vi "Current_and_Spectrum_View_new.vi"() -> ()   [LabVIEW 2009]
doc: "I. Description:\nThis example demonstrates how to perform an analog software triggered acquisition. The example allows the user to specify the triggering condition and the number of pre-trigger samples to acquire.\n \nII. Instructions for Running:\n1. Select the physical channel to correspond to where your signal is input on the DAQ device.\n2. Enter the minimum and maximum voltage ranges.\nNote: For better accuracy try to match the Input Ranges to the expected voltage level of the measured signal.\n3. Specify the rate of the sample clock. \n4. Specify the number of samples to read per iteration of the continuous input operation. These samples will then be monitored for the trigger condition. The trigger condition is determined by the parameters explained below.\n5. Specify the index of the channel that will be monitored for the requested condition. The first channel in the scan list will have an index equals to 0. It's possible to verify the name of the selected channel once the VI is run, after setting the Channel Index value.\n6. Set the triggering condition to be applied to the channel specified by the Channel Index value. The conditions created for this example are:\n\n- Rising Edge: The trigger condition is met as soon as the monitored signal falls below the Hysteresis window and then crosses past the specified Level.\n- Falling Edge: The trigger condition is met as soon as the monitored signal rises above the Hysteresis window and then crosses past the specified Level.\n- Above Level: The trigger condition is met as soon as the monitored signal is above the specified Level. \n- Below Level: The trigger condition is met as soon as the monitored signal is below the specified Level.\n- When Inside Window: The trigger condition is met as soon as the monitored signal is within the specified window.\n- When Outside Window: The trigger condition is met as soon as the monitored signal is not within the specified window.\n\n7. Set the Level value to be used by the selected condition.\n8. Set the Window Amplitude/ Hysteresis to be used by the Window/Edge conditions\n\n- The upper limit of the conditional window is calculated by adding the Window Amplitude to the condition Level.\n- The lower limit of the conditional window is calculated by subtracting the Window Amplitude from the condition Level.\n- The Hysteresis window for the Rising Edge condition is defined as Level minus the Hysteresis value. \n- The Hysteresis window for the Falling Edge condition is defined as Level plus the Hysteresis value.\n\n8. Set the number of pre-trigger samples if desired.\n\nIII. Block Diagram Steps:\n1. Create an analog input voltage channel.\n2. Find out how many channels are being used in this operation.\n3. Define the Sample Clock Rate. Additionally, define the sample mode to be continuous.\n4. Show the Channel Name of the Condition Channel.\n5. Initialize the data arrays to be used for holding successive iterations of data. This pre-allocation of memory improves the performance of the application. Refer to the VI documentation for more information.\n\nNOTE: The number of samples that meet the triggering condition is not fixed; it depends on the value of the monitored signal. This means that the number of samples to be returned by Analog Trigger Through Software (Scaled).VI may vary from one iteration to the next. In order to avoid dynamically allocating memory while filtering the data (a process that creates), this example pre-allocates arrays for the data before the acquisition starts. The arrays are initialized to the maximum number of elements expected per iteration.\n\n6. Call the Start VI to start the acquisition.\n7. Read the scaled analog input data.\nNote: The Shift Registers attached to the While Loop are used to keep track of triggering status and previous data samples (needed for pre-triggered acquisitions). \n8. Use the Analog Trigger Through Software (Scaled).VI specifically created for this example to detect the requested trigger condition through software.\n9. Show the acquired data if the trigger condition is met.\n10. Stop the loop if the trigger condition is met, an error occurs or the Stop button is pressed. \n11. Call the Clear Task VI to clear the Task.\n12. Use the popup dialog box to display an error or warning if any.\n\nIV. I/O Connections Overview:\nMake sure your signal input terminal matches the Physical Channel I/O control. For further connection information, refer to your hardware reference manual."
uses:
  <vilib>/Utility/error.llb/DialogType.ctl
  <vilib>/DAQmx/configure/timing.llb/DAQmx Timing (Sample Clock).vi
  <vilib>/DAQmx/create/channels.llb/DAQmx Create Channel (AI-Voltage-Basic).vi
  <vilib>/DAQmx/read.llb/DAQmx Read (Analog 2D DBL NChan NSamp).vi
  <vilib>/express/express analysis/Spectral/XNode/ExpressSpectralMeasurementsBlockNode.xnode
  <vilib>/express/express analysis/Spectral/Block/exnSpectralBlock spectral measurements peak poly.vi
  <vilib>/express/express analysis/Spectral/Block/exnSpectralBlock spectral measurements peak DDT.vi
  <vilib>/Utility/file.llb/Write To Spreadsheet File (DBL).vi
panel:
  in  "Save?":bool
  in  "Path":path
  in  "SAVED FILES":i32
  in  "Filename":string
  out "x/y":dbl[](array[numeric])
  out "Waveform Graph 2":dynamicdata(graph)
  out "# Pretrigger Samples\nAcquired":i32
  out "Waveform Graph":dbl[][](graph)
  out "Pre-Trigger Error Indicator":bool caption="Error Indicator\n(Indicates if trigger occurs before\npre-trigger samples were acquired)"
  in  "Pretrigger Samples":i32
  in  "Window Amplitude":dbl=0.5 caption="Window Amplitude\n/Hysteresis" step=0.10000000149011612 format="%.2p"
  out "Channel Name":string
  in  "Condition":T1(ring)=enum."Above Level"
  in  "Channel Index":i32
  in  "Level":dbl=-11.0 step=0.10000000149011612 format="%.2p"
  in  "Samples to Read":i32=40000 caption="Samples to Read per Iteration"
  in  "Maximum Value":dbl=10.0 format="%.2p"
  in  "Minimum Value":dbl=-10.0 format="%.2p"
  in  "Physical Channel":tag="Dev1/ai0"
  in  "Rate":dbl=10000.0 caption="Sample Rate (Hz)" format="%0.2f"
  in  "Stop":bool caption="stop"
  # "For instructions, select Help>>Show Context Help"
  # "Channel Parameters"
  # "Timing Parameters"
  # "Triggering Parameters"
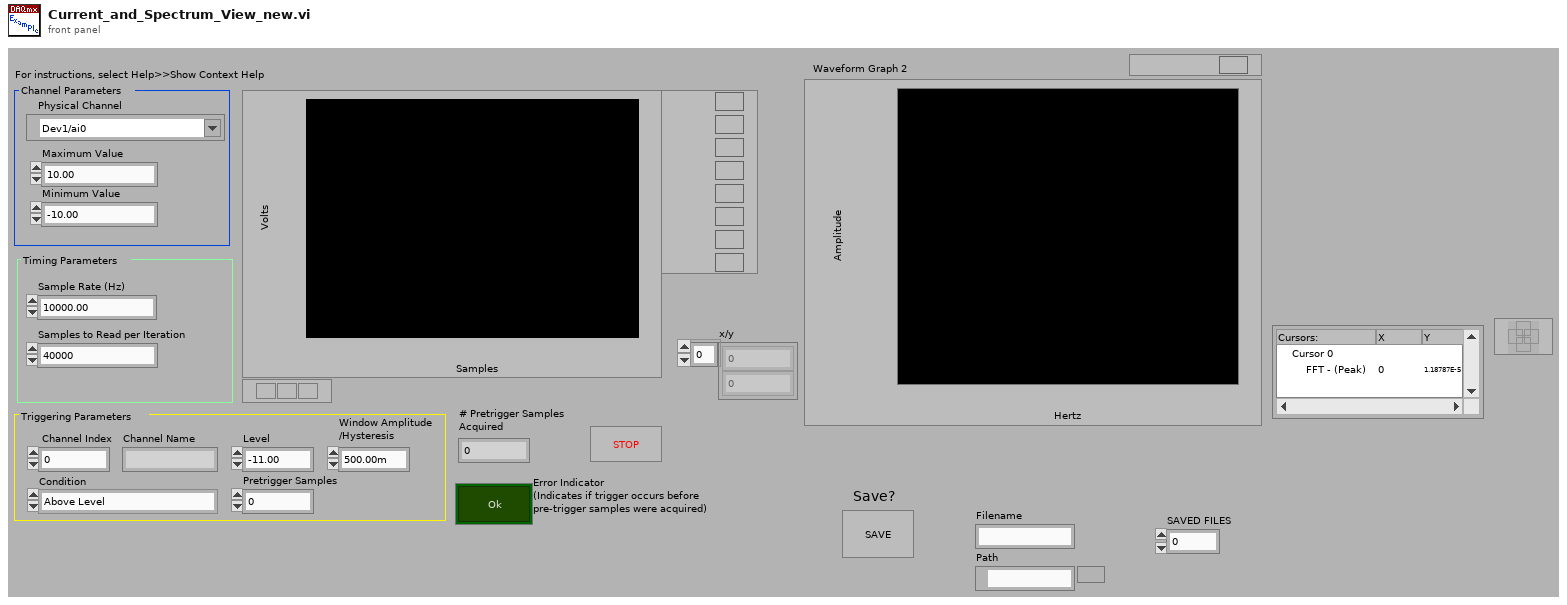
[diagram p1: front panel]
types:
  T1 = enum16{"Rising Edge", "Falling Edge", "Above Level", "Below Level", "When Inside Window", "When Outside Window"}
  T2 = typedef "DialogType.ctl" = u16
  T3 = cluster{"averaging mode":u16, "weighting mode":u16, "number of averages":u32}
  T4 = cluster{"dB On (F)":bool, "unwrap phase (F)":bool, "convert to degree (F)":bool}
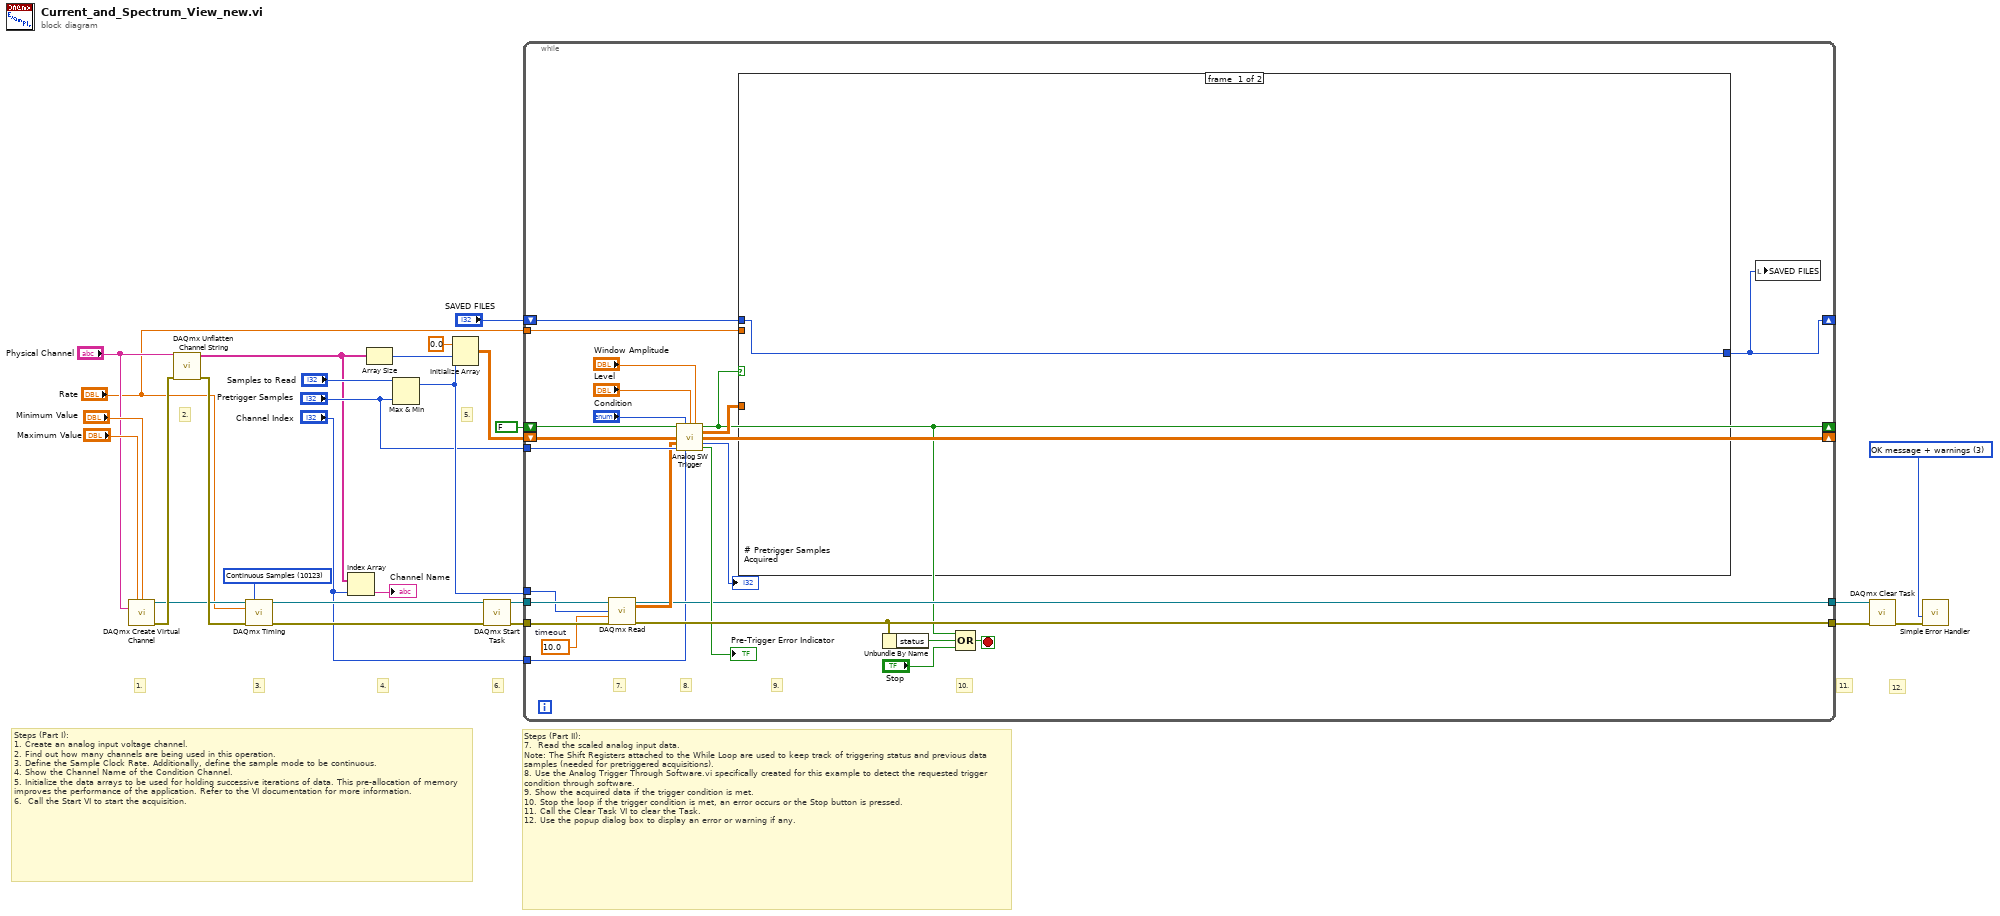
[diagram p0: block diagram]
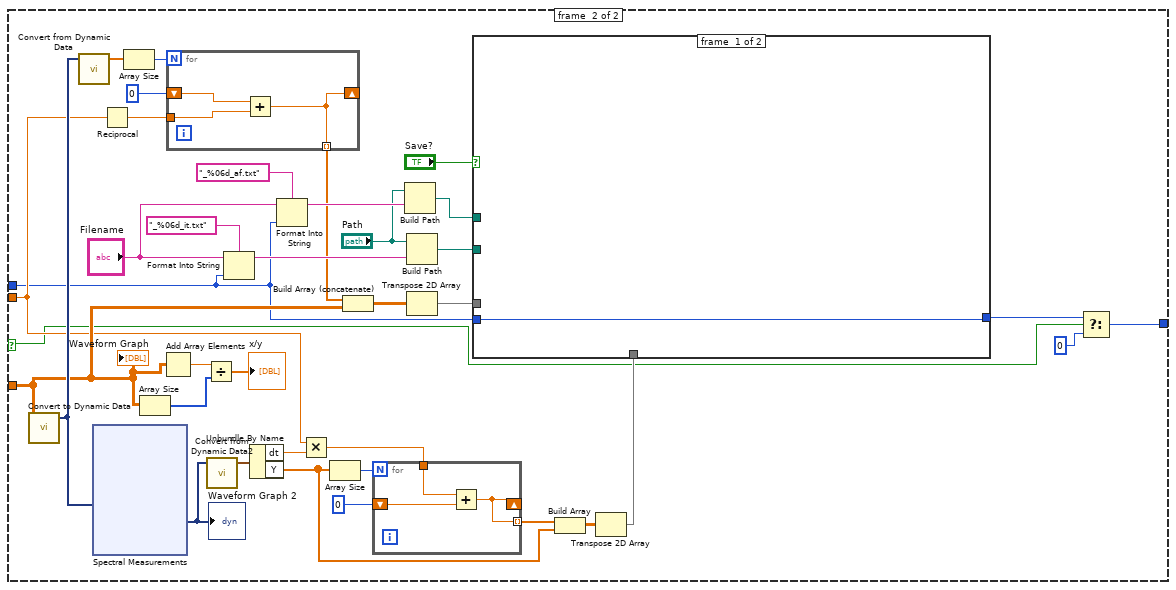
[diagram p2: hidden frame]
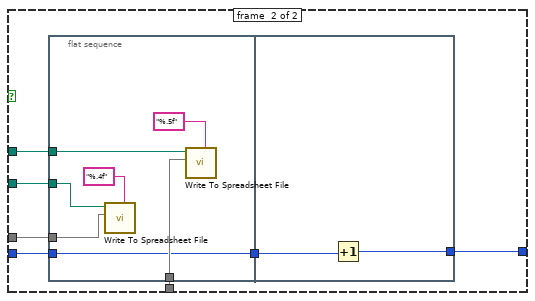
[diagram p3: hidden frame]
diagram:
  w21 = T2 3 items=["no dialog", "OK message", "continue or stop message", "OK message + warnings", "continue/stop + warnings"] ("type of dialog (OK msg:1)")
  w22 = 10123 items=["Finite Samples"=10178, "Continuous Samples"=10123] ("sample mode")
  # "5."
  # "3."
  # "Steps (Part II): \n7.  Read the scaled analog input data.\nNote: The Shift Registers attached to the While Loop are used to keep track of triggering status and previous data samples (needed for pretriggered acquisitions). \n8. Use the Analog Trigger Through Software.vi specifically created for this example to detect the requested trigger condition through software.\n9. Show the acquired data if the trigger condition is met.\n10. Stop the loop if the trigger condition is met, an error occurs or the Stop button is pressed. \n11. Call the Clear Task VI to clear the Task.\n12. Use the popup dialog box to display an error or warning if any."
  # "4."
  # "12."
  # "Steps (Part I): \n1. Create an analog input voltage channel.\n2. Find out how many channels are being used in this operation.\n3. Define the Sample Clock Rate. Additionally, define the sample mode to be continuous.\n4. Show the Channel Name of the Condition Channel.\n5. Initialize the data arrays to be used for holding successive iterations of data. This pre-allocation of memory improves the performance of the application. Refer to the VI documentation for more information.\n6.  Call the Start VI to start the acquisition."
  # "11."
  # "6."
  # "2."
  # "1."
  n1 = call-poly <vilib>:"DAQmx Create Virtual Channel.vi"("maximum value"="Maximum Value", "minimum value"="Minimum Value", "physical channels"="Physical Channel") -> ("task out"=w11:refnum<k21>, "error out"=w16:errorcluster)  [unwired: 11 in]
  n2 = call <vilib>:"DAQmx Unflatten Channel String.vi"("names in"="Physical Channel", "error in"=w16) -> ("names out"=w10:string[], "error out"=w15:errorcluster)  [unwired: 12 in]
  n3 = call-poly <vilib>:"DAQmx Timing.vi"("task/channels in"=w11, "sample mode"=w22, "rate"="Rate", "error in"=w15) -> ("task out"=w7:refnum<k21>, "error out"=w8:errorcluster)  [unwired: 10 in]
  n4 = Index Array(array=w10, index="Channel Index") -> (element=→"Channel Name":string)
  n5 = Array Size(array=w10) -> (size(s)=w4:i32)
  n6 = Max & Min(x="Samples to Read", y="Pretrigger Samples") -> (max(x,y)=w13:i32)  [unwired: 1 out]
  n7 = Initialize Array(0.0, w4, w13) -> (w17:dbl[][])
  n8 = call <vilib>:"DAQmx Start Task.vi"("task/channels in"=w7, "error in"=w8) -> ("task out"=w23:refnum<k21>, "error out"=w25:errorcluster)  [unwired: 12 in]
  n9 = while {
    tunnel: w25 -> [w52]
    tunnel: [w51] -> w19
    tunnel: w23 -> [w50]
    tunnel: [w33] -> w20
    tunnel: w13 -> [w48]
    shift-right: [w31] -> _
    shift-left: FALSE ("stop") -> [w47]
    shift-right: [w36] -> _
    shift-left: w17 -> [w37]
    tunnel: "Pretrigger Samples" -> [w40]
    tunnel: "Channel Index" -> [w32]
    tunnel: "Rate" -> [w30]
    shift-right: [w28] -> _
    shift-left: "SAVED FILES" -> [w29]
    stop <- w42 stop-if-true
    w49 = 10.0  # timeout
    # "10."
    # "9."
    # "7."
    # "8."
    n10 = call-poly <vilib>:"DAQmx Read.vi"("task/channels in"=w50, "number of samples per channel"=w48, "timeout"=w49, "error in"=w52) -> ("task out"=w33:refnum<k21>, "data"=w38:dbl[][], "error out"=w51:errorcluster)  [unwired: 9 in]
    n11 = call "Analog SW Trigger.vi"("Triggered?"=w47, "Condition"="Condition", "Level"="Level", "Window Amplitude"="Window Amplitude", "Initialized Data Array"=w37, "Input Raw Data"=w38, "Pretrigger Samples"=w40, "Index of Condition Channel"=w32) -> ("Trigger Out"=w31:bool, "Output Data (Scaled)"=w35:dbl[][], "Raw Data Out"=w36:dbl[][], "# Pretrigger Samples"=→"# Pretrigger Samples\nAcquired":i32, "Pre-Trigger Error"=→"Pre-Trigger Error Indicator":bool)  [unwired: 3 in]
    n12 = case shown="True" w31 {
      selector: w31 -> [_ w56]
      tunnel: w35 -> [_ w74]
      tunnel: w30 -> [_ w67]
      tunnel: w29 -> [w53 w58]
      tunnel: [w53 w54] -> w28
      frame #0 {
      }
      frame #1 {
        n13 = call "Convert to Dynamic Data"("2D Array"=w74) -> ("Dynamic Data Type"=w80:dynamicdata)  [unwired: 3 in]
        n14 = call "Convert from Dynamic Data"("Dynamic Data Type"=w80) -> ("Array"=w79:dbl[])  [unwired: 3 in]
        n15 = xnode "Spectral Measurements"("Signals"=w80) -> ("FFT - (Peak)"=w72:dynamicdata)  [unwired: 1 in, 2 out]
        "Waveform Graph 2" <- w72
        n16 = Reciprocal(x=w67) -> (1/x=w78:dbl)
        n17 = Array Size(array=w79) -> (size(s)=w81:i32)
        n18 = Array Size(array=w74) -> (size(s)=w89:i32[])
        n19 = Add Array Elements(numeric array=w74) -> (sum=w90:dbl)
        n20 = for {
          N: w81 -> [_]
          tunnel: w78 -> [w113]
          shift-right: [w111] -> _
          shift-left: 0 -> [w112]
          tunnel: [w111] -> w76 mode=indexing
          n21 = Add(x=w112, y=w113) -> (x+y=w111:dbl)
        }
        n22 = Divide(x=w90, y=w89) -> (x/y=→"x/y":dbl[])
        n23 = call "Convert from Dynamic Data2"("Dynamic Data Type"=w72) -> ("Waveform"=w71:waveform(dbl))  [unwired: 3 in]
        n24 = Format Into String(format string="_%06d_it.txt", initial string="Filename", w58) -> (resulting string=w82:string)  [unwired: 1 in, 1 out]
        n25 = Unbundle By Name(w71) -> ("dt"=w68:dbl, "Y"=w64:dbl[])
        n26 = Format Into String(format string="_%06d_af.txt", initial string="Filename", w58) -> (resulting string=w84:string)  [unwired: 1 in, 1 out]
        n27 = Multiply(x=w67, y=w68) -> (x*y=w66:dbl)
        n28 = Array Size(array=w64) -> (size(s)=w70:i32)
        n29 = Build Array (concatenate)(w76, w74) -> (w75:dbl[][])
        n30 = for {
          N: w70 -> [_]
          shift-right: [w91] -> _
          shift-left: 0 -> [w93]
          tunnel: w66 -> [w92]
          tunnel: [w91] -> w65 mode=indexing
          n31 = Add(x=w92, y=w93) -> (x+y=w91:dbl)
        }
        n32 = Build Path(base path="Path", name or relative path=w84) -> (appended path=w59:path)
        n33 = Build Path(base path="Path", name or relative path=w82) -> (appended path=w61:path)
        n34 = Transpose 2D Array(2D array=w75) -> (transposed array=w62:dbl[][])
        n35 = Build Array(w65, w64) -> (w63:dbl[][])
        n36 = Transpose 2D Array(2D array=w63) -> (transposed array=w60:dbl[][])
        n37 = case shown="True" "Save?" {
          tunnel: w62 -> [_ w101]
          tunnel: w61 -> [_ w100]
          tunnel: w60 -> [_ w99]
          tunnel: w59 -> [_ w98]
          tunnel: w58 -> [w94 w96]
          tunnel: [w94 w95] -> w57
          frame #0 {
          }
          frame #1 {
            n38 = flat-sequence {
              tunnel: w101 -> [w103]
              tunnel: w100 -> [w108]
              tunnel: w99 -> [w106]
              tunnel: w98 -> [w105]
              tunnel: [w102] -> w97
              tunnel: w96 -> [w102]
              tunnel: w97 -> [w110]
              tunnel: [w109] -> w95
              frame #0 {
                n39 = call-poly <vilib>:"Write To Spreadsheet File.vi"("format (%.3f)"="%.4f", "2D data"=w103, "file path (dialog if empty)"=w108) -> ()  [unwired: 5 in, 1 out]
                n40 = call-poly <vilib>:"Write To Spreadsheet File.vi"("format (%.3f)"="%.5f", "2D data"=w106, "file path (dialog if empty)"=w105) -> ()  [unwired: 5 in, 1 out]
              }
              frame #1 {
                n41 = Increment(x=w110) -> (x+1=w109:i32)
              }
            }
          }
        }
        n42 = Select(t=w57, s=w56, f=0) -> (s? t:f=w54:i32)
        "Waveform Graph" <- w74
      }
    }
    n43 = Unbundle By Name(w51) -> ("status"=w43:bool)
    n44 = Compound Arithmetic op=OR(w31, w43, "Stop") -> (w42:bool)
    n45 = local write "SAVED FILES"(w28) -> ()
  }
  n46 = call <vilib>:"DAQmx Clear Task.vi"("task in"=w20, "error in"=w19) -> ("error out"=w24:errorcluster)  [unwired: 13 in]
  n47 = call <vilib>:"Simple Error Handler.vi"("type of dialog (OK msg:1)"=w21, "error in (no error)"=w24) -> ()  [unwired: 3 in, 5 out]
